vi "Verify Simple Smith Plot.vi"(1 "[user-specified font]":T1={"Font Name:"="Current Font", "Size"=36, "Strikeout?"=FALSE, "Italic?"=FALSE, "Underline?"=FALSE, "Outline?"=TRUE, "Shadow?"=TRUE, "Bold?"=TRUE}, 2 "desired font(Application)":T2(ring), 3 "Text To Draw":string) -> (0 "Smith Plot":picture)   [LabVIEW 2013]
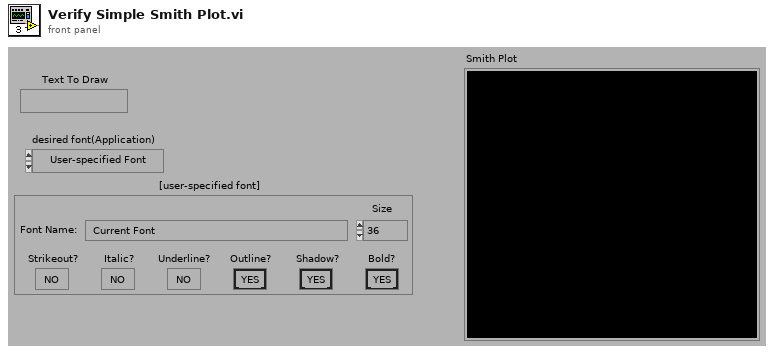
[diagram p1: front panel]
types:
  T1 = cluster{"Font Name:":string, "Size":i16, "Strikeout?":bool, "Italic?":bool, "Underline?":bool, "Outline?":bool, "Shadow?":bool, "Bold?":bool}
  T2 = enum16{"User-specified Font", "Application Font", "System Font", "Dialog Font"}
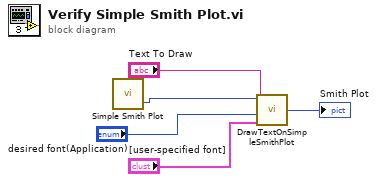
[diagram p0: block diagram]
diagram:
  n1 = call "Simple Smith Plot.vi"() -> ("Pict Out"=w5:picture)  [unwired: 6 out]
  n2 = call "DrawTextOnSimpleSmithPlot.vi"("Pict In"=w5, "Text To Draw"="Text To Draw", "desired font(Application)"="desired font(Application)", "[user-specified font]"="[user-specified font]") -> ("Pict Out"=→"Smith Plot":picture)  [unwired: 1 out]
